vi "NI OCR-OCR.vi"(8 "error in":errorcluster, 11 "Buffer Data In":T1={"VI Refnum"=refnum, "Src Image"=refnum, "Dst Image"=refnum, "Ctl Refnum []"=[], "Ctl Label"=[], "User Event"=refnum, "Event Registration Refnum"=refnum, "Timeout"=0, "IMAQ OCR Session"=refnum, "Objects"=[], "ROI Descriptor"={"Global Rectangle"=[], "Contours"=[]}, "Settings"={"Objects"=0, "Threshold"=128, "Reject Border"=FALSE, "Fill Holes"=FALSE, "Min Object Size"=FALSE, "Min Size"=3, "Max Object Size"=FALSE, "Max Size"=100, "Show Search Area"=FALSE, "Show Center"=TRUE, "Show Bounding Box"=TRUE}} {"Settings"."Objects" items=["Bright Objects", "Dark Objects"]; "Settings"."Threshold" min=1 max=999999999 step=1; "Settings"."Max Size" min=1 max=999999999 step=1; "Settings"."Min Size" min=1 max=999999999 step=1; "ROI Descriptor"."Contours"."Type" items=["No Selection", "Point", "Line", "Rectangle", "Oval", "Polygon", "Freehand Region", "Annulus", "Unused2", "Unused3", "Broken Line", "Freehand Line", "Rotated Rectangle"]; "Objects"."Aspect Ratio" format="%.2f"; "Objects"."Orientation" format="%.2f"; "Objects"."Area" format="%.2f"; "Objects"."Object Center"."Y" format="%.2f"; "Objects"."Object Center"."X" format="%.2f"}) -> (0 "error out":errorcluster, 3 "Buffer Data Out":T1={"VI Refnum"=refnum, "Src Image"=refnum, "Dst Image"=refnum, "Ctl Refnum []"=[], "Ctl Label"=[], "User Event"=refnum, "Event Registration Refnum"=refnum, "Timeout"=0, "IMAQ OCR Session"=refnum, "Objects"=[], "ROI Descriptor"={"Global Rectangle"=[], "Contours"=[]}, "Settings"={"Objects"=0, "Threshold"=128, "Reject Border"=FALSE, "Fill Holes"=FALSE, "Min Object Size"=FALSE, "Min Size"=3, "Max Object Size"=FALSE, "Max Size"=100, "Show Search Area"=FALSE, "Show Center"=TRUE, "Show Bounding Box"=TRUE}} {"Settings"."Objects" items=["Bright Objects", "Dark Objects"]; "Settings"."Threshold" min=1 max=999999999 step=1; "Settings"."Max Size" min=1 max=999999999 step=1; "Settings"."Min Size" min=1 max=999999999 step=1; "ROI Descriptor"."Contours"."Type" items=["No Selection", "Point", "Line", "Rectangle", "Oval", "Polygon", "Freehand Region", "Annulus", "Unused2", "Unused3", "Broken Line", "Freehand Line", "Rotated Rectangle"]; "Objects"."Aspect Ratio" format="%.2f"; "Objects"."Orientation" format="%.2f"; "Objects"."Area" format="%.2f"; "Objects"."Object Center"."Y" format="%.2f"; "Objects"."Object Center"."X" format="%.2f"})   [LabVIEW 2016]
uses:
  Data Def/NI OCR-Buffer Data.ctl
  <vilib>/vision/Image Controls.llb/IMAQ Image.ctl
  Data Def/NI OCR-User Event Data.ctl
  <vilib>/vision/OCR.llb/IMAQ OCR Session.ctl
  <vilib>/vision/NI_Vision_Development_Module.lvlib
panel:
  out "x-y":u32
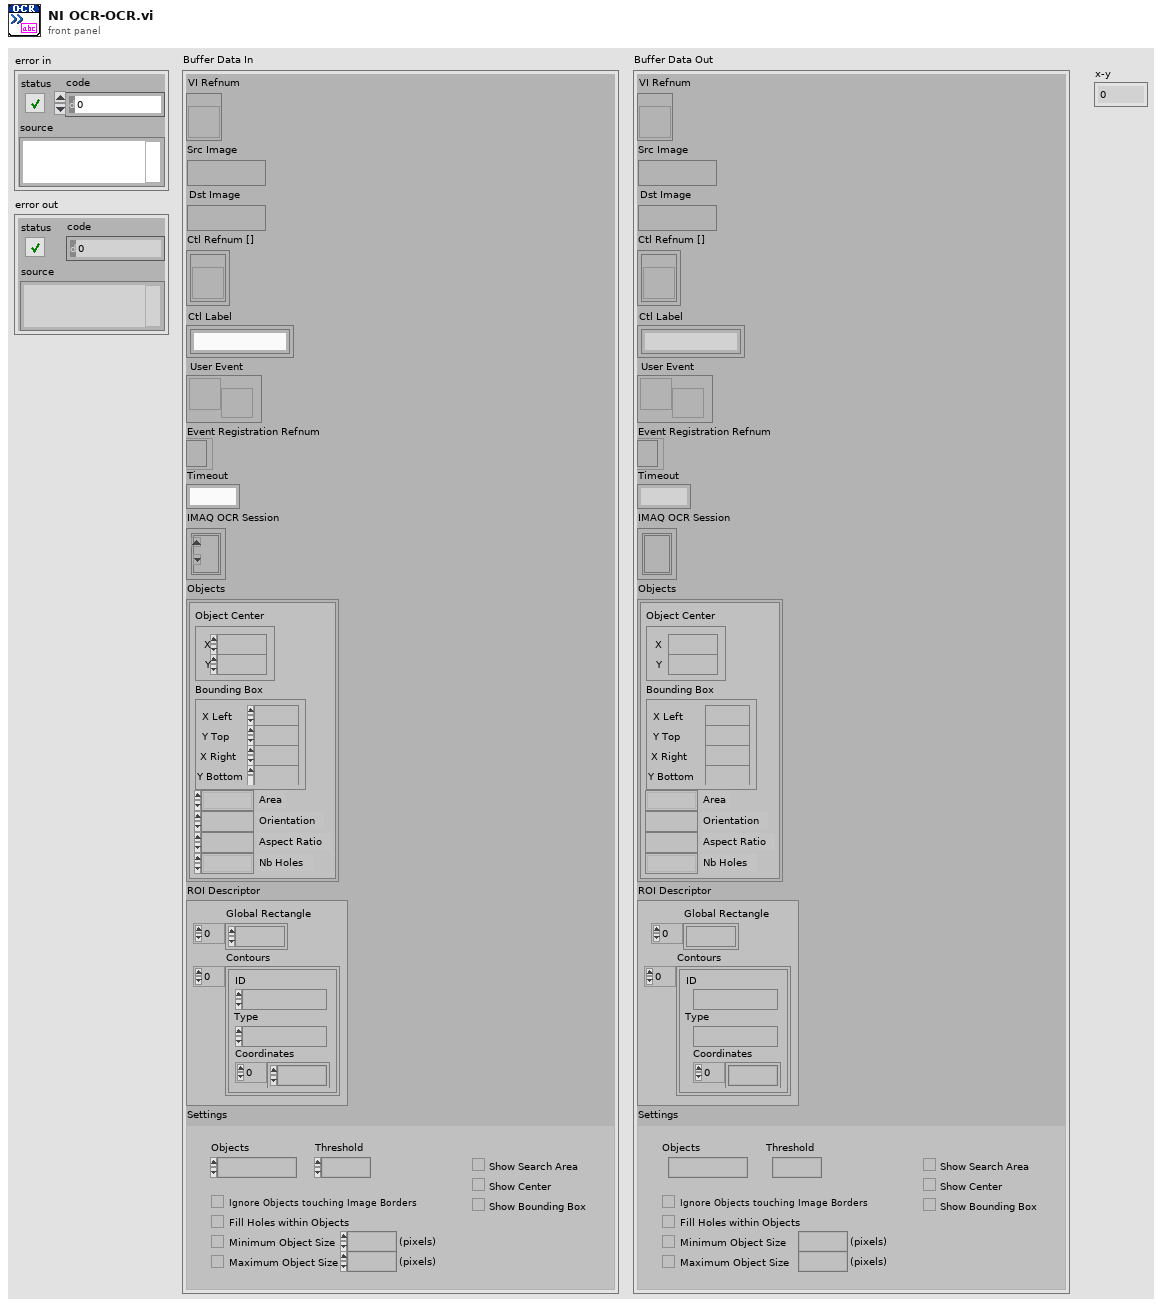
[diagram p1: front panel]
types:
  T1 = typedef "NI OCR-Buffer Data.ctl" = cluster{"VI Refnum":refnum<vi>, "Src Image":T2, "Dst Image":T2, "Ctl Refnum []":refnum<vi>[], "Ctl Label":string[], "User Event":refnum<user-event>, "Event Registration Refnum":refnum<event-registration>, "Timeout":i32, "IMAQ OCR Session":T3, "Objects":cluster{"Object Center":cluster{"X":sgl, "Y":sgl}, "Bounding Box":cluster{"X Left":i32, "Y Top":i32, "X Right":i32, "Y Bottom":i32}, "Area":sgl, "Orientation":sgl, "Aspect Ratio":sgl, "Nb Holes":i32}[], "ROI Descriptor":T4, "Settings":cluster{"Objects":u16, "Threshold":i32, "Reject Border":bool, "Fill Holes":bool, "Min Object Size":bool, "Min Size":i32, "Max Object Size":bool, "Max Size":i32, "Show Search Area":bool, "Show Center":bool, "Show Bounding Box":bool}}
  T2 = typedef "IMAQ Image.ctl" = refnum<image>
  T3 = typedef "IMAQ OCR Session.ctl" = refnum<k1>
  T4 = typedef "ROI Descriptor" = cluster{"Global Rectangle":i32[], "Contours":cluster{"ID":enum32{"External", "Internal"}, "Type":u32, "Coordinates":i32[]}[]}
  T5 = cluster{"Objects":u16, "Threshold":i32, "Reject Border":bool, "Fill Holes":bool, "Min Object Size":bool, "Min Size":i32, "Max Object Size":bool, "Max Size":i32, "Show Search Area":bool, "Show Center":bool, "Show Bounding Box":bool}
  T6 = typedef "IMAQ Rectangle" = cluster{"Left":i32, "Top":i32, "Right":i32, "Bottom":i32, "Rotation":dbl}
  T7 = cluster{"Object Center":cluster{"X":sgl, "Y":sgl}, "Bounding Box":cluster{"X Left":i32, "Y Top":i32, "X Right":i32, "Y Bottom":i32}, "Area":sgl, "Orientation":sgl, "Aspect Ratio":sgl, "Nb Holes":i32}[]
  T8 = cluster{"Desired Font (Application)":enum16{"User-specified Font", "Application Font", "System Font", "Dialog Font"}, "[User-specified Font]":cluster{"Font Name":string, "Size":i16, "Strikeout?":bool, "Italic?":bool, "Underline?":bool, "Outline?":bool, "Shadow?":bool, "Bold?":bool, "Rotation Angle":dbl}, "Horizontal Alignment":i16, "Vertical Alignment":i16}
  T9 = cluster{"X Left":i32, "Y Top":i32, "X Right":i32, "Y Bottom":i32}
  T10 = typedef "IMAQ OCR Character Report 2.ctl" = cluster{"Character Value":string, "Classification Score":i32, "Verification Score":i32, "Verified":bool, "Character Statistics":cluster{"Threshold Range":cluster{"Lower value":sgl, "Upper value":sgl}, "Left Offset":i32, "Top Offset":i32, "Width":i32, "Height":i32, "Character Size":i32}}
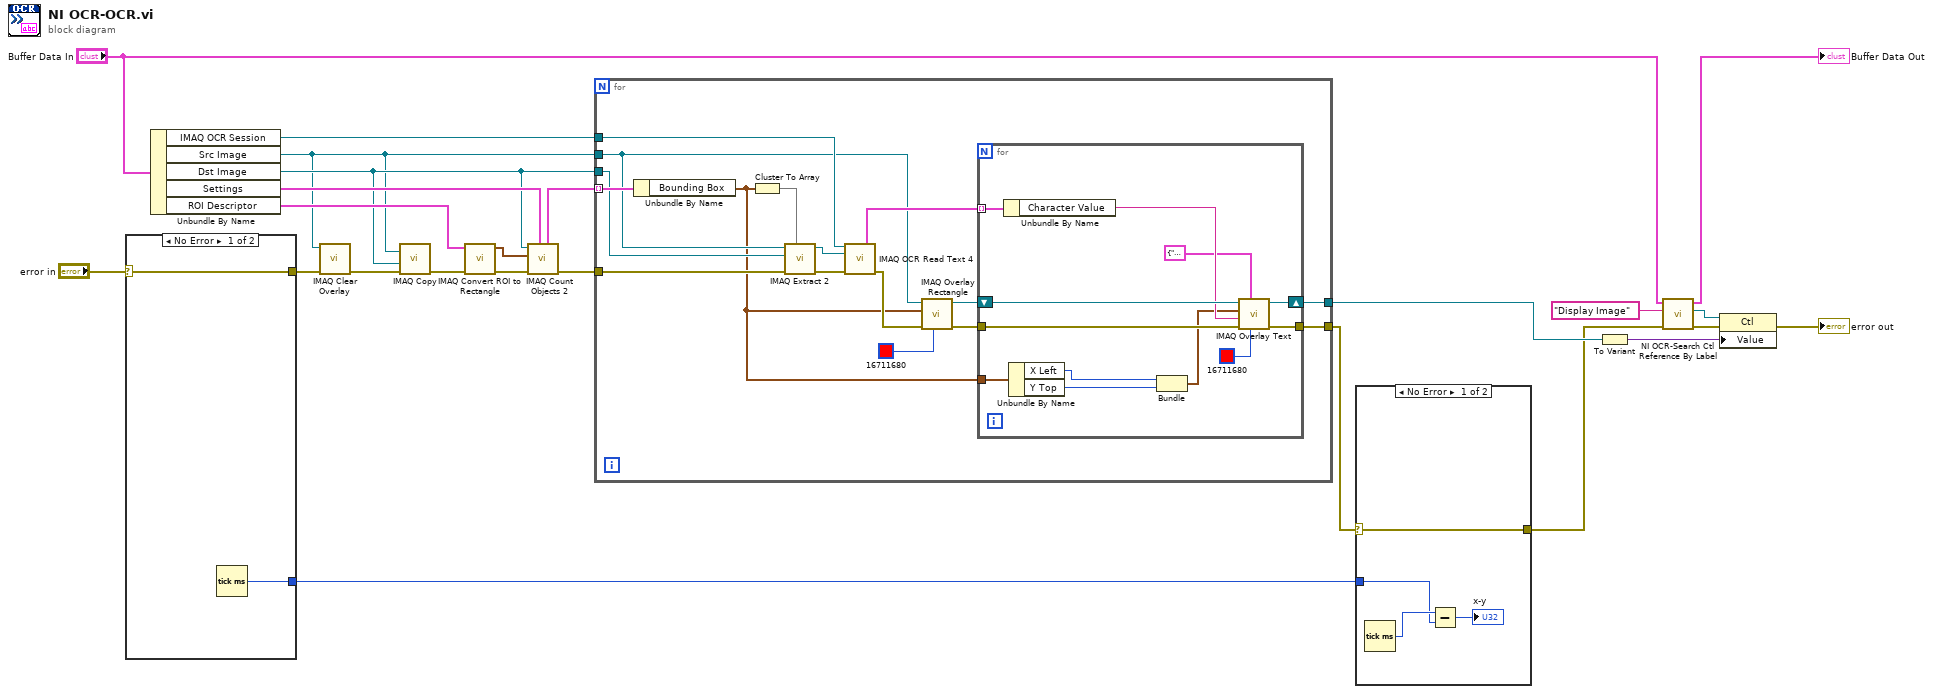
[diagram p0: block diagram]
diagram:
  n1 = case shown="No Error" "error in" {
    selector: "error in" -> [w26 _]
    tunnel: [w26 _] -> w3
    tunnel: [w25 _] -> w4
    frame No Error {
      n2 = Tick Count (ms)() -> (millisecond timer value=w25:u32)
    }
    frame Error {
    }
  }
  n3 = Unbundle By Name("Buffer Data In") -> ("IMAQ OCR Session"=w20:T3, "Src Image"=w1:T2, "Dst Image"=w8:T2, "Settings"=w11:T5, "ROI Descriptor"=w12:T4)
  n4 = call "IMAQ Clear Overlay"("error in (no error)"=w3, "Image"=w1) -> ("error out"=w2:errorcluster)  [unwired: 8 in, 1 out]
  n5 = call "IMAQ Copy"("error in (no error)"=w2, "Image Dst"=w8, "Image Src"=w1) -> ("error out"=w13:errorcluster)  [unwired: 3 in, 1 out]
  n6 = call "IMAQ Convert ROI to Rectangle"("error in (no error)"=w13, "ROI Descriptor"=w12) -> ("error out"=w15:errorcluster, "Rectangle"=w16:T6)  [unwired: 7 in]
  n7 = call "IMAQ Count Objects 2"("Settings"=w11, "error in (no error)"=w15, "Search Rect (entire image)"=w16, "Image"=w8) -> ("error out"=w9:errorcluster, "Objects"=w10:T7)  [unwired: 3 in, 3 out]
  n8 = for {
    tunnel: w20 -> [w42]
    tunnel: [w37] -> w6
    tunnel: [w36] -> w17
    tunnel: w10 -> [w33] mode=indexing
    tunnel: w9 -> [w34]
    tunnel: w1 -> [w29]
    tunnel: w8 -> [w32]
    n9 = Unbundle By Name(w33) -> ("Bounding Box"=w27:T9)
    n10 = Cluster To Array(cluster=w27) -> (array=w35:i32[])
    n11 = call "IMAQ Extract 2"("Optional Rectangle"=w35, "error in (no error)"=w34, "Image Dst"=w32, "Image Src"=w29) -> ("error out"=w31:errorcluster, "Image Dst Out"=w30:T2)  [unwired: 6 in]
    n12 = call "IMAQ OCR Read Text 4"("IMAQ OCR Session"=w42, "Image"=w30, "error in (no error)"=w31) -> ("Character Reports"=w38:T10[], "error out"=w41:errorcluster)  [unwired: 6 in, 5 out]
    n13 = call "IMAQ Overlay Rectangle"("Color"=u32 16711680, "error in (no error)"=w41, "Rectangle"=w27, "Image"=w29) -> ("error out"=w40:errorcluster, "Image Out"=w39:T2)  [unwired: 6 in]
    n14 = for {
      tunnel: w40 -> [w53]
      tunnel: w38 -> [w54] mode=indexing
      tunnel: [w51] -> w37
      shift-right: [w50] -> w36
      shift-left: w39 -> [w52]
      tunnel: w27 -> [w45]
      n15 = Unbundle By Name(w54) -> ("Character Value"=w49:string)
      n16 = Unbundle By Name(w45) -> ("X Left"=w43:i32, "Y Top"=w44:i32)
      n17 = Bundle("X Left"=w43, "Y Top"=w44) -> (w46:cluster{"X Left":i32, "Y Top":i32})  [unwired: 1 in]
      n18 = call "IMAQ Overlay Text"("Text Color (black)"=u32 16711680, "Font, Size & Style"=T8 {"Desired Font (Application)"=enum."User-specified Font", "[User-specified Font]"={"Font Name"="", "Size"=12, "Strikeout?"=FALSE, "Italic?"=FALSE, "Underline?"=FALSE, "Outline?"=FALSE, "Shadow?"=FALSE, "Bold?"=FALSE, "Rotation Angle"=0.0}, "Horizontal Alignment"=0, "Vertical Alignment"=0}, "error in (no error)"=w53, "String"=w49, "Origin"=w46, "Image"=w52) -> ("error out"=w51:errorcluster, "Image Out"=w50:T2)  [unwired: 4 in]
    }
  }
  n19 = case shown="No Error" w6 {
    selector: w6 -> [w58 w59]
    tunnel: [w58 w59] -> w5
    tunnel: w4 -> [w56 _]
    frame No Error {
      n20 = Tick Count (ms)() -> (millisecond timer value=w57:u32)
      n21 = Subtract(x=w57, y=w56) -> (x-y=→"x-y":u32)
    }
    frame Error {
    }
  }
  n22 = To Variant(anything=w17) -> (Variant=w21:variant)
  n23 = call "NI OCR-Search Ctl Reference By Label.vi"("error in"=w5, "Ctl Label"="Display Image", "Buffer Data In"="Buffer Data In") -> ("error out"=w23:errorcluster, "Ctl Refnum"=w22:refnum<vi>, "Buffer Data Out"=→"Buffer Data Out":T1)  [unwired: 5 in, 1 out]
  n24 = property class="Ctl"(reference=w22, error in=w23, "Value"=w21) -> (error out=→"error out":errorcluster)  [unwired: 1 out]
